vi "Get Monitor.Values All.vi"(8 "error in":errorcluster) -> (0 "error out":errorcluster, 3 "Signal Data":waveform(dbl)[](array[waveform]))   [LabVIEW 2021, in "XNET-CAN-Signal-Logger.lvlib"]
uses:
  XNET-CAN-Signal-Logger.lvlib
  Global Variables.vi
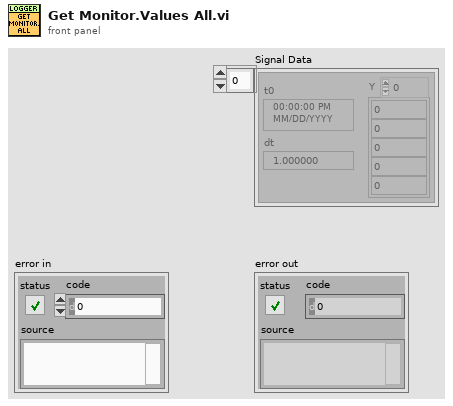
[diagram p1: front panel]
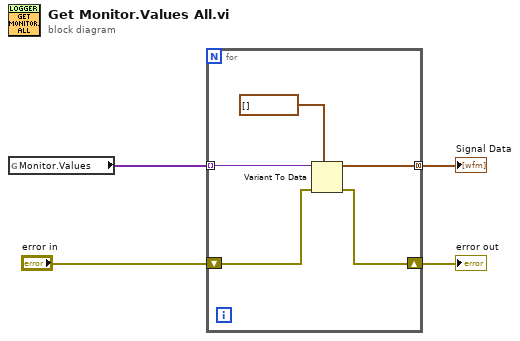
[diagram p0: block diagram]
diagram:
  n1 = global read "Global Variables.vi" "Monitor.Values"() -> (w4:variant[])
  n2 = for {
    tunnel: w4 -> [w9] mode=indexing
    tunnel: [w8] -> w1 mode=concatenating
    shift-right: [w6] -> w2
    shift-left: "error in" -> [w7]
    n3 = Variant To Data(error in=w7, type=waveform(dbl)[] [] ("Data"), Variant=w9) -> (data=w8:waveform(dbl)[], error out=w6:errorcluster)
  }
  "error out" <- w2
  "Signal Data" <- w1
